vi "Apply Shunts.vi"(8 "error in (no error)":errorcluster, 11 "VISA Refnum in":refnum<visa-resource-name>) -> (0 "error out":errorcluster)   [LabVIEW 2018]
uses:
  Agilent 34970/Agilent 34970.lvlib
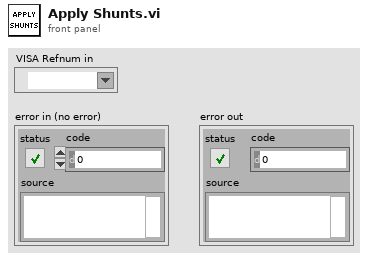
[diagram p1: front panel]
types:
  T1 = enum16{"None", "XON / XOFF", "RTS / CTS", "DTR / DSR"}
  T2 = cluster{"Timeout Value (10000)":u32, "Baud Rate (57600)":enum16{"1200", "2400", "4800", "9600", "19200", "38400", "57600", "115200"}, "Flow Control (1:XON/XOFF)":enum16{"None", "XON / XOFF", "RTS / CTS", "DTR / DSR"}}
  T3 = enum16{"1200", "2400", "4800", "9600", "19200", "38400", "57600", "115200"}
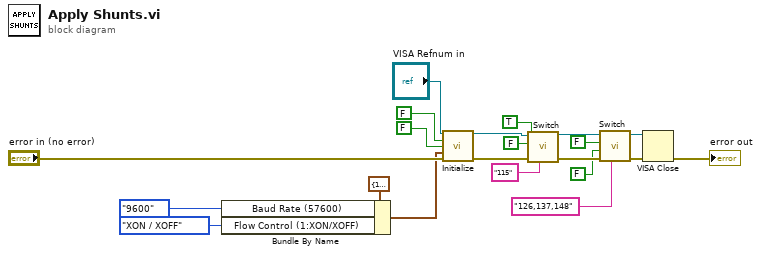
[diagram p0: block diagram]
diagram:
  n1 = Bundle By Name(cluster=T2 {"Timeout Value (10000)"=10000, "Baud Rate (57600)"=enum."9600", "Flow Control (1:XON/XOFF)"=enum."XON / XOFF"} ("Serial Port Configuration"), "Baud Rate (57600)"=T3."9600", "Flow Control (1:XON/XOFF)"=T1."XON / XOFF") -> (w10:T2)
  n2 = call "Initialize.vi"("VISA Resource Name"="VISA Refnum in", "ID Query (T: Check)"=FALSE, "Reset (T: Reset)"=FALSE, "Serial Port Configuration"=w10, "error in (no error)"="error in (no error)") -> ("VISA Resource Name Out"=w16:refnum<visa-resource-name>, "error out"=w15:errorcluster)  [unwired: 9 in]
  n3 = call "Switch.vi"("Channel List(empty)"="115", "error in (no error)"=w15, "Close Exclusive (F:Normal)"=TRUE, "Open/Close (F:Close)"=FALSE, "VISA Resource Name"=w16) -> ("error out"=w8:errorcluster, "VISA Resource Name Out"=w7:refnum<visa-resource-name>)  [unwired: 4 in, 1 out]
  n4 = call "Switch.vi"("Channel List(empty)"="126,137,148", "error in (no error)"=w8, "Close Exclusive (F:Normal)"=FALSE, "Open/Close (F:Close)"=FALSE, "VISA Resource Name"=w7) -> ("error out"=w17:errorcluster, "VISA Resource Name Out"=w18:refnum<visa-resource-name>)  [unwired: 4 in, 1 out]
  n5 = VISA Close(VISA resource name=w18, error in (no error)=w17) -> (error out=→"error out":errorcluster)
